vi "Config Source Event.vi"(6 "Input Event":string="0", 8 "error in":errorcluster, 9 "Channel (Channel A)":T1, 10 "Node In":string, 11 "VISA resource name":refnum<visa-resource-name>) -> (0 "error out":errorcluster, 2 "Node Out":string, 3 "VISA resource name out":refnum<visa-resource-name>, 4 "Command String":string)   [LabVIEW 2012, in "Keithley 2600 Series.lvlib"]
doc: "This VI configures the source event in the advanced trigger model.\n\n<b>Functions and Attributes Used</b>\nsmuX.trigger.source.sequence.count\nsmuX.trigger.source.sequence.number\nsmuX.trigger.source.stimulus"
uses:
  Keithley 2600 Series.lvlib
  Private/GlobalVariables.vi
  Channel.ctl
panel:
  # "(c) 2008 Keithley Instruments, Inc.  ALL RIGHTS RESERVED."
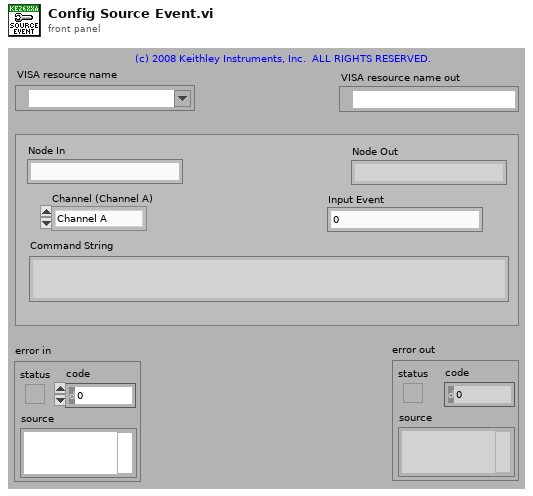
[diagram p1: front panel]
types:
  T1 = typedef "Keithley 2600 Series.lvlib/Channel.ctl" = enum32{"Channel A", "Channel B"}
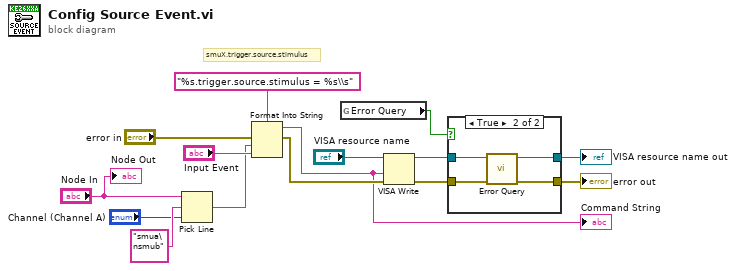
[diagram p0: block diagram]
diagram:
  # "smuX.trigger.source.stimulus"
  n1 = Pick Line(string ("")="Node In", multi-line string="smua\nsmub", line index="Channel (Channel A)") -> (output string=w2:string)
  n2 = Format Into String(format string="%s.trigger.source.stimulus = %s\\s", error in="error in", w2, "Input Event") -> (resulting string=w3:string, error out=w10:errorcluster)  [unwired: 1 in]
  "Command String" <- w3
  n3 = global read "GlobalVariables.vi" "Error Query"() -> (w8:bool)
  n4 = VISA Write(VISA resource name="VISA resource name", write buffer=w3, error in (no error)=w10) -> (VISA resource name out=w7:refnum<visa-resource-name>, error out=w6:errorcluster)  [unwired: 1 out]
  n5 = case shown="True" w8 {
    tunnel: w7 -> [w17 w21]
    tunnel: w6 -> [w16 w20]
    tunnel: [w17 w19] -> w5
    tunnel: [w16 w18] -> w4
    frame False {
    }
    frame True {
      n6 = call "Error Query.vi"("error in (no error)"=w20, "VISA resource name"=w21) -> ("error out"=w18:errorcluster, "VISA resource name out"=w19:refnum<visa-resource-name>)  [unwired: 8 out]
    }
  }
  "VISA resource name out" <- w5
  "error out" <- w4
  "Node Out" <- "Node In"
